vi "Filtered analysis.vi"() -> (5 "Plug in titles":string[](array[string]), 7 "Plug in values":string[](array[string]))   [LabVIEW 2011]
uses:
  <vilib>/Analysis/3filter.llb/Filter Passband Type.ctl
  Globals/Meas_global.vi
  <vilib>/Analysis/3filter.llb/Zero Phase Filter (Cascade, DBL).vi
  <vilib>/Analysis/NI_AALBase.lvlib
panel:
  out "XY Graph 5":cluster{"Time (ms)":dbl[], "Eng Values":dbl[]}[](graph)
  in  "Cutoff frequency (Hz)":dbl=50.0
  out "uw/u'w'":dbl
  out "u^2 4":dbl
  out "U 4":dbl
  out "u^2 3":dbl
  out "U 3":dbl
  out "XY Graph 4":cluster{"Time (ms)":dbl[], "Eng Values":dbl[]}[](graph)
  out "XY Graph 3":cluster{"Time (ms)":dbl[], "Eng Values":dbl[]}[](graph)
  out "uw/u'w' Filtered":dbl
  out "u^2 Filtered":dbl
  out "U filtered":dbl
  out "u^2 filtered":dbl
  out "U filtered":dbl
  in  "Invert values?":bool
  in  "Filter 2nd Instrument data?":bool
  in  "Freq Cutoff Inst 2":dbl=100.0
  in  "Freq Cutoff Inst 1":dbl=100.0
  in  "Filter 1st Instrument Data?":bool
  out "Time for max corr coeff":dbl
  out "Max corr coeff":dbl
  in  "Start point":dbl
  in  "Time step":dbl
  in  "Input own variables?":bool=TRUE
  out "Inst name 2":string
  out "Inst name":string
  out "Start point":dbl
  out "XY Graph 2":cluster{dbl[], dbl[]}(graph)
  out "Time step":dbl
  in  "Number of estimates":i32
  out "XY Graph":cluster{"Time (ms)":dbl[], "Eng Values":dbl[]}[](graph)
  in  "Instrumnt 2":i32=1
  in  "Instrument 1":i32
  # "Time lag"
  # "Correlation"
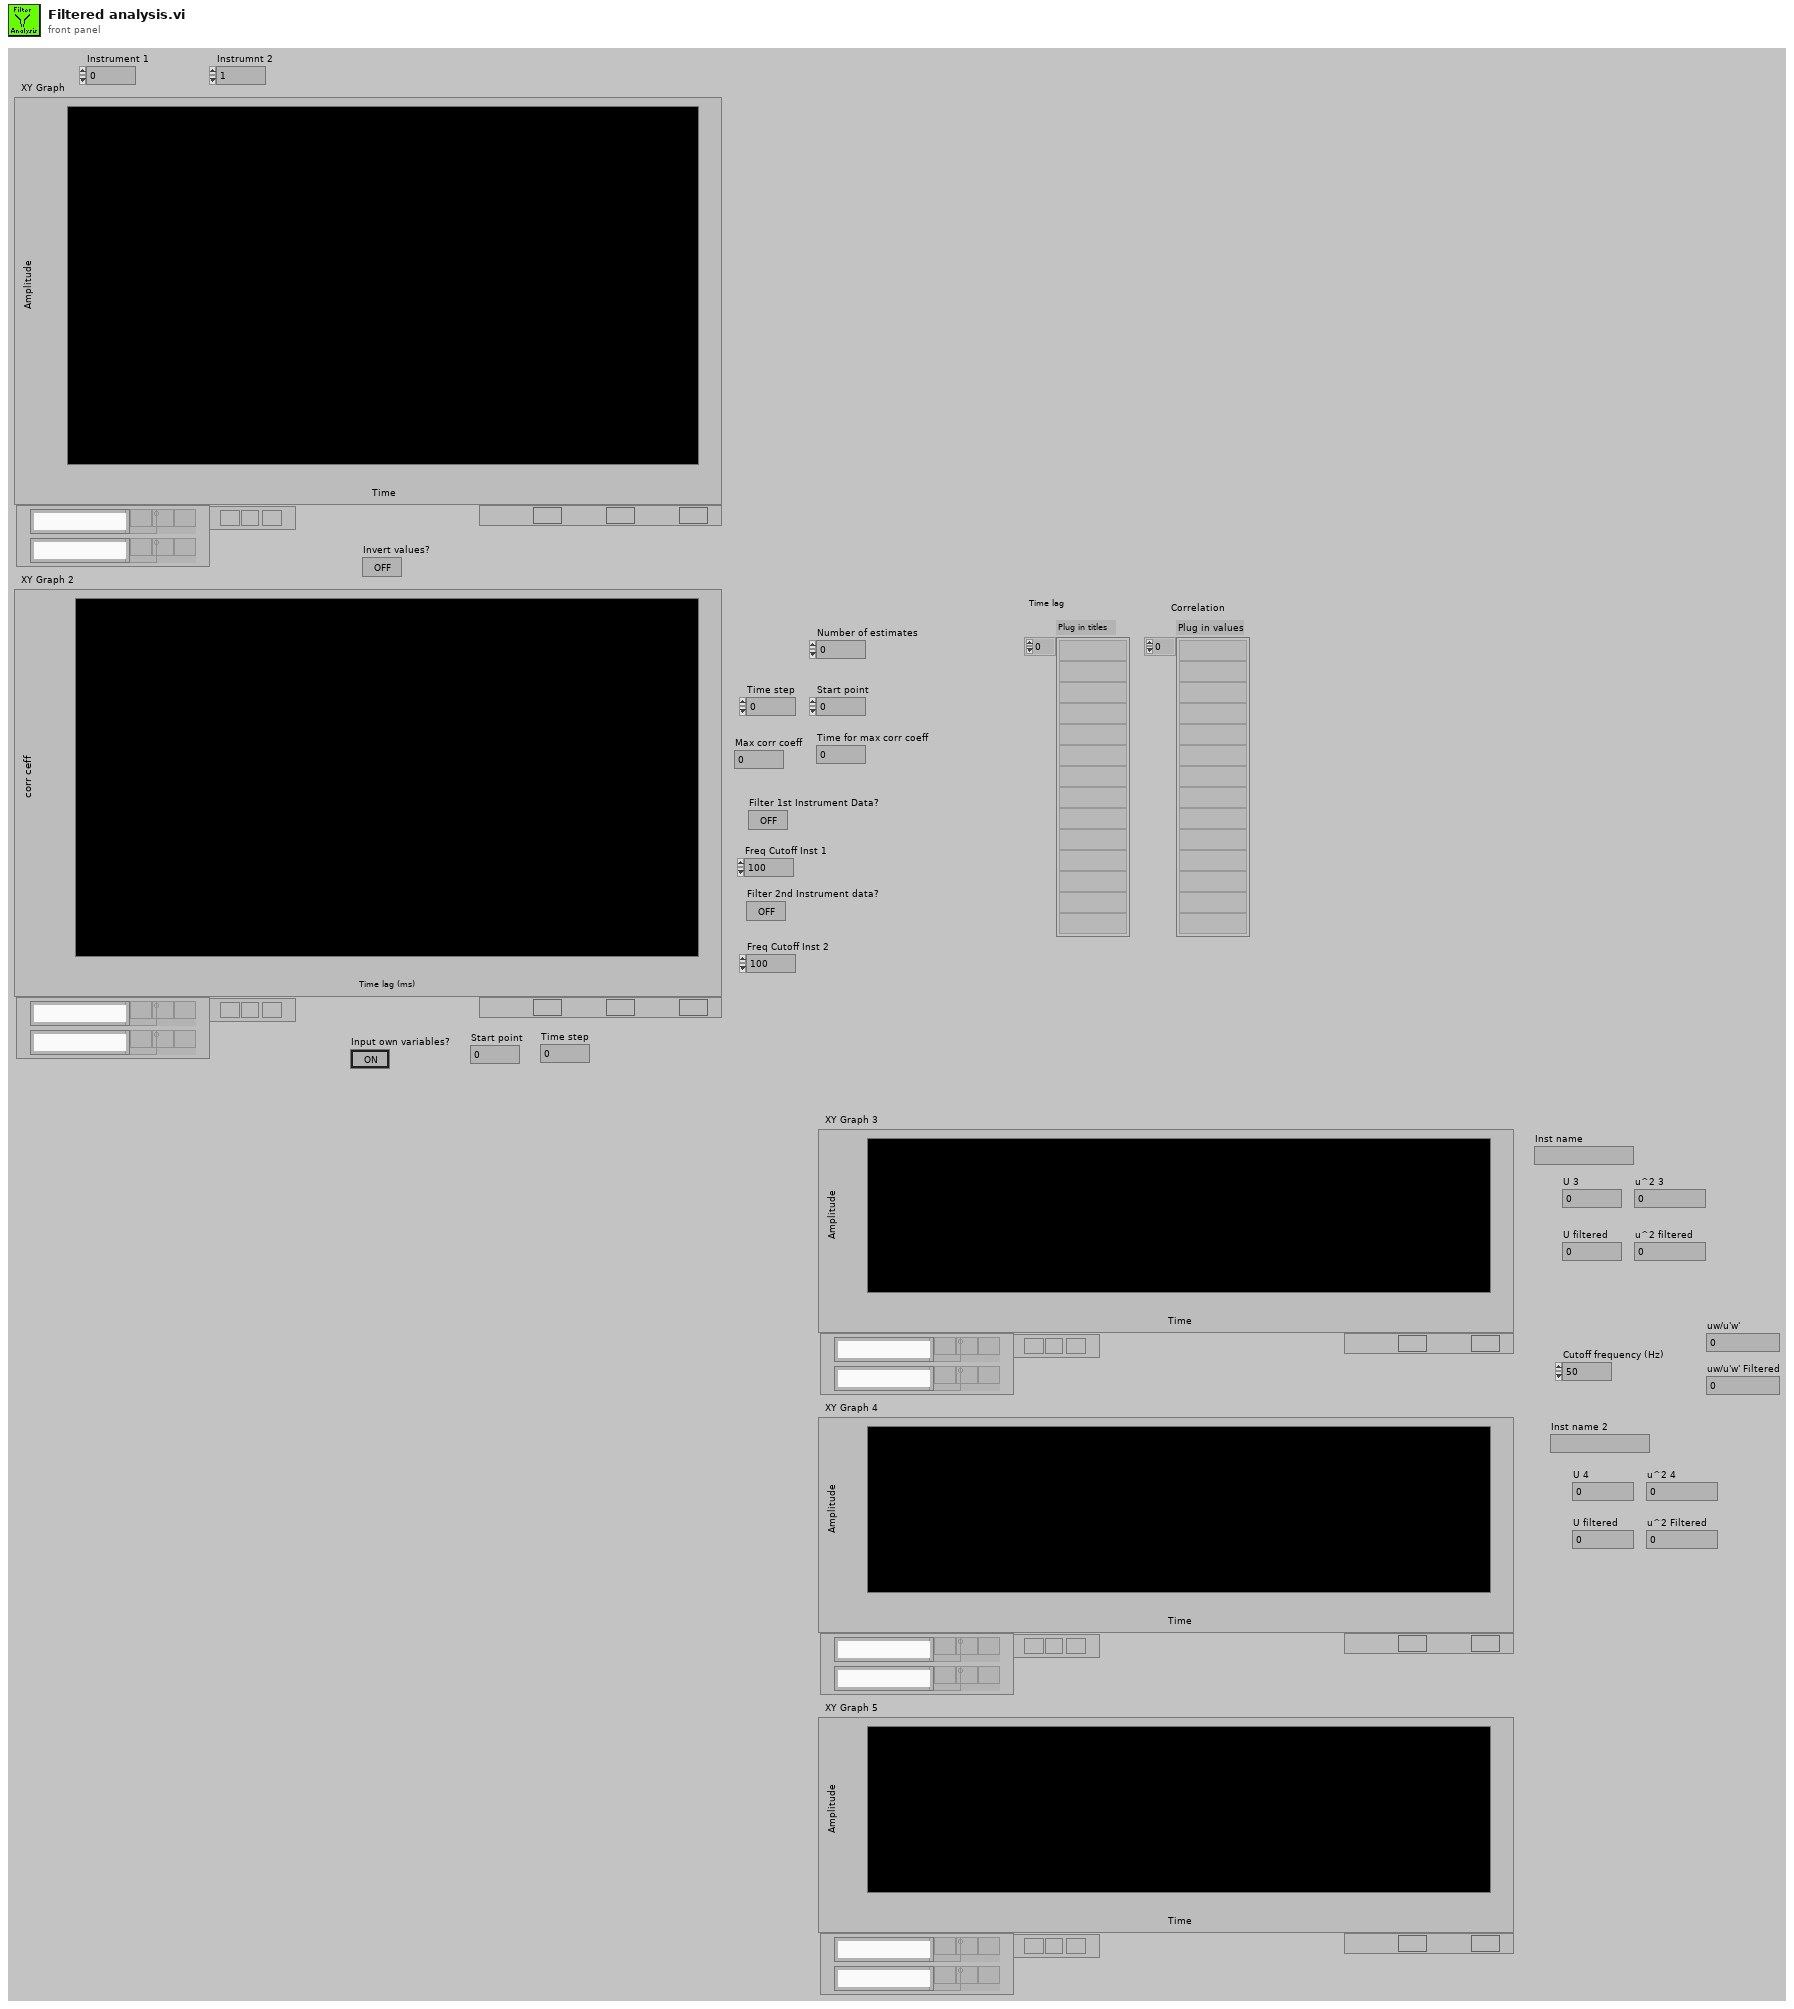
[diagram p1: front panel]
types:
  T1 = typedef "Analysis_info_cluster.ctl" = cluster{"Colour":u32, "Inst type":T2, "Inst name":string, "Symbol":string, "Code name":string, "Extra Info":string, "Inst Array":T3, "Extra Titles":string[], "Extra Values":string[], "Eng Values":dbl[], "Time (ms)":dbl[], "Voltage":dbl[], "U":dbl, "u^2":dbl, "u^3":dbl, "u^4":dbl, "Skew_u":dbl, "Kurt_u":dbl, "Sd Error in Mean":dbl, "% u'/U":dbl, "X":dbl, "Y":dbl, "Z":dbl, "Spectra":T4, "Autocorrelation":T4, "Timescale integral to 25%":dbl, "Sd Error in Variance":dbl, "Calib File":path, "Calib Constants":dbl[], "Histogram":T4, "Output Position":bool, "Full Stats":bool, "Weighting":dbl[], "Av Sampling Rate":dbl, "Av No of Samples":dbl, "Total Meas Time (s)":dbl}
  T2 = typedef "Inst_type.ctl" = enum16{"Propeller anemometer", "Raw voltage", "Pressure Transducer", "Pitot-static tube", "Preston tube", "Hot wire", "Cross wire 1", "Cross wire 2", "Generic Linear", "Generic Polynomial", "Generic BackPoly", "Fast FID", "Thermocouple", "Cold wire", "Pulsed Wire", "LDA Vel", "LDA Tran time", "LDA Arr time"}
  T3 = typedef "Instrument_Array.ctl" = enum16{"PWA", "LDA", "Analogue"}
  T4 = typedef "XY_Plot_Cluster.ctl" = cluster{"First Name":string, "Second Name":string, "X axis name":string, "Y axis name":string, "X array":dbl[], "Y array":dbl[]}
  T5 = typedef "NI_AALBase.lvlib/Filter Passband Type.ctl" = enum32{"Lowpass", "Highpass", "Bandpass", "Bandstop"}
  T6 = cluster{"filter structure":enum32{"IIR 2nd Order", "IIR 4th Order"}, "Reverse Coefficients":dbl[], "Forward Coefficients":dbl[]}
  T7 = typedef "Correlation_cluster1.ctl" = cluster{"U inst":string, "uw":dbl, "u^2w":dbl, "uw^2":dbl, "uw/u'w'":dbl, "W inst":string, "uw^3":dbl, "u^3w":dbl, "u^2w^2":dbl, "Index U":i32, "Index W":i32}
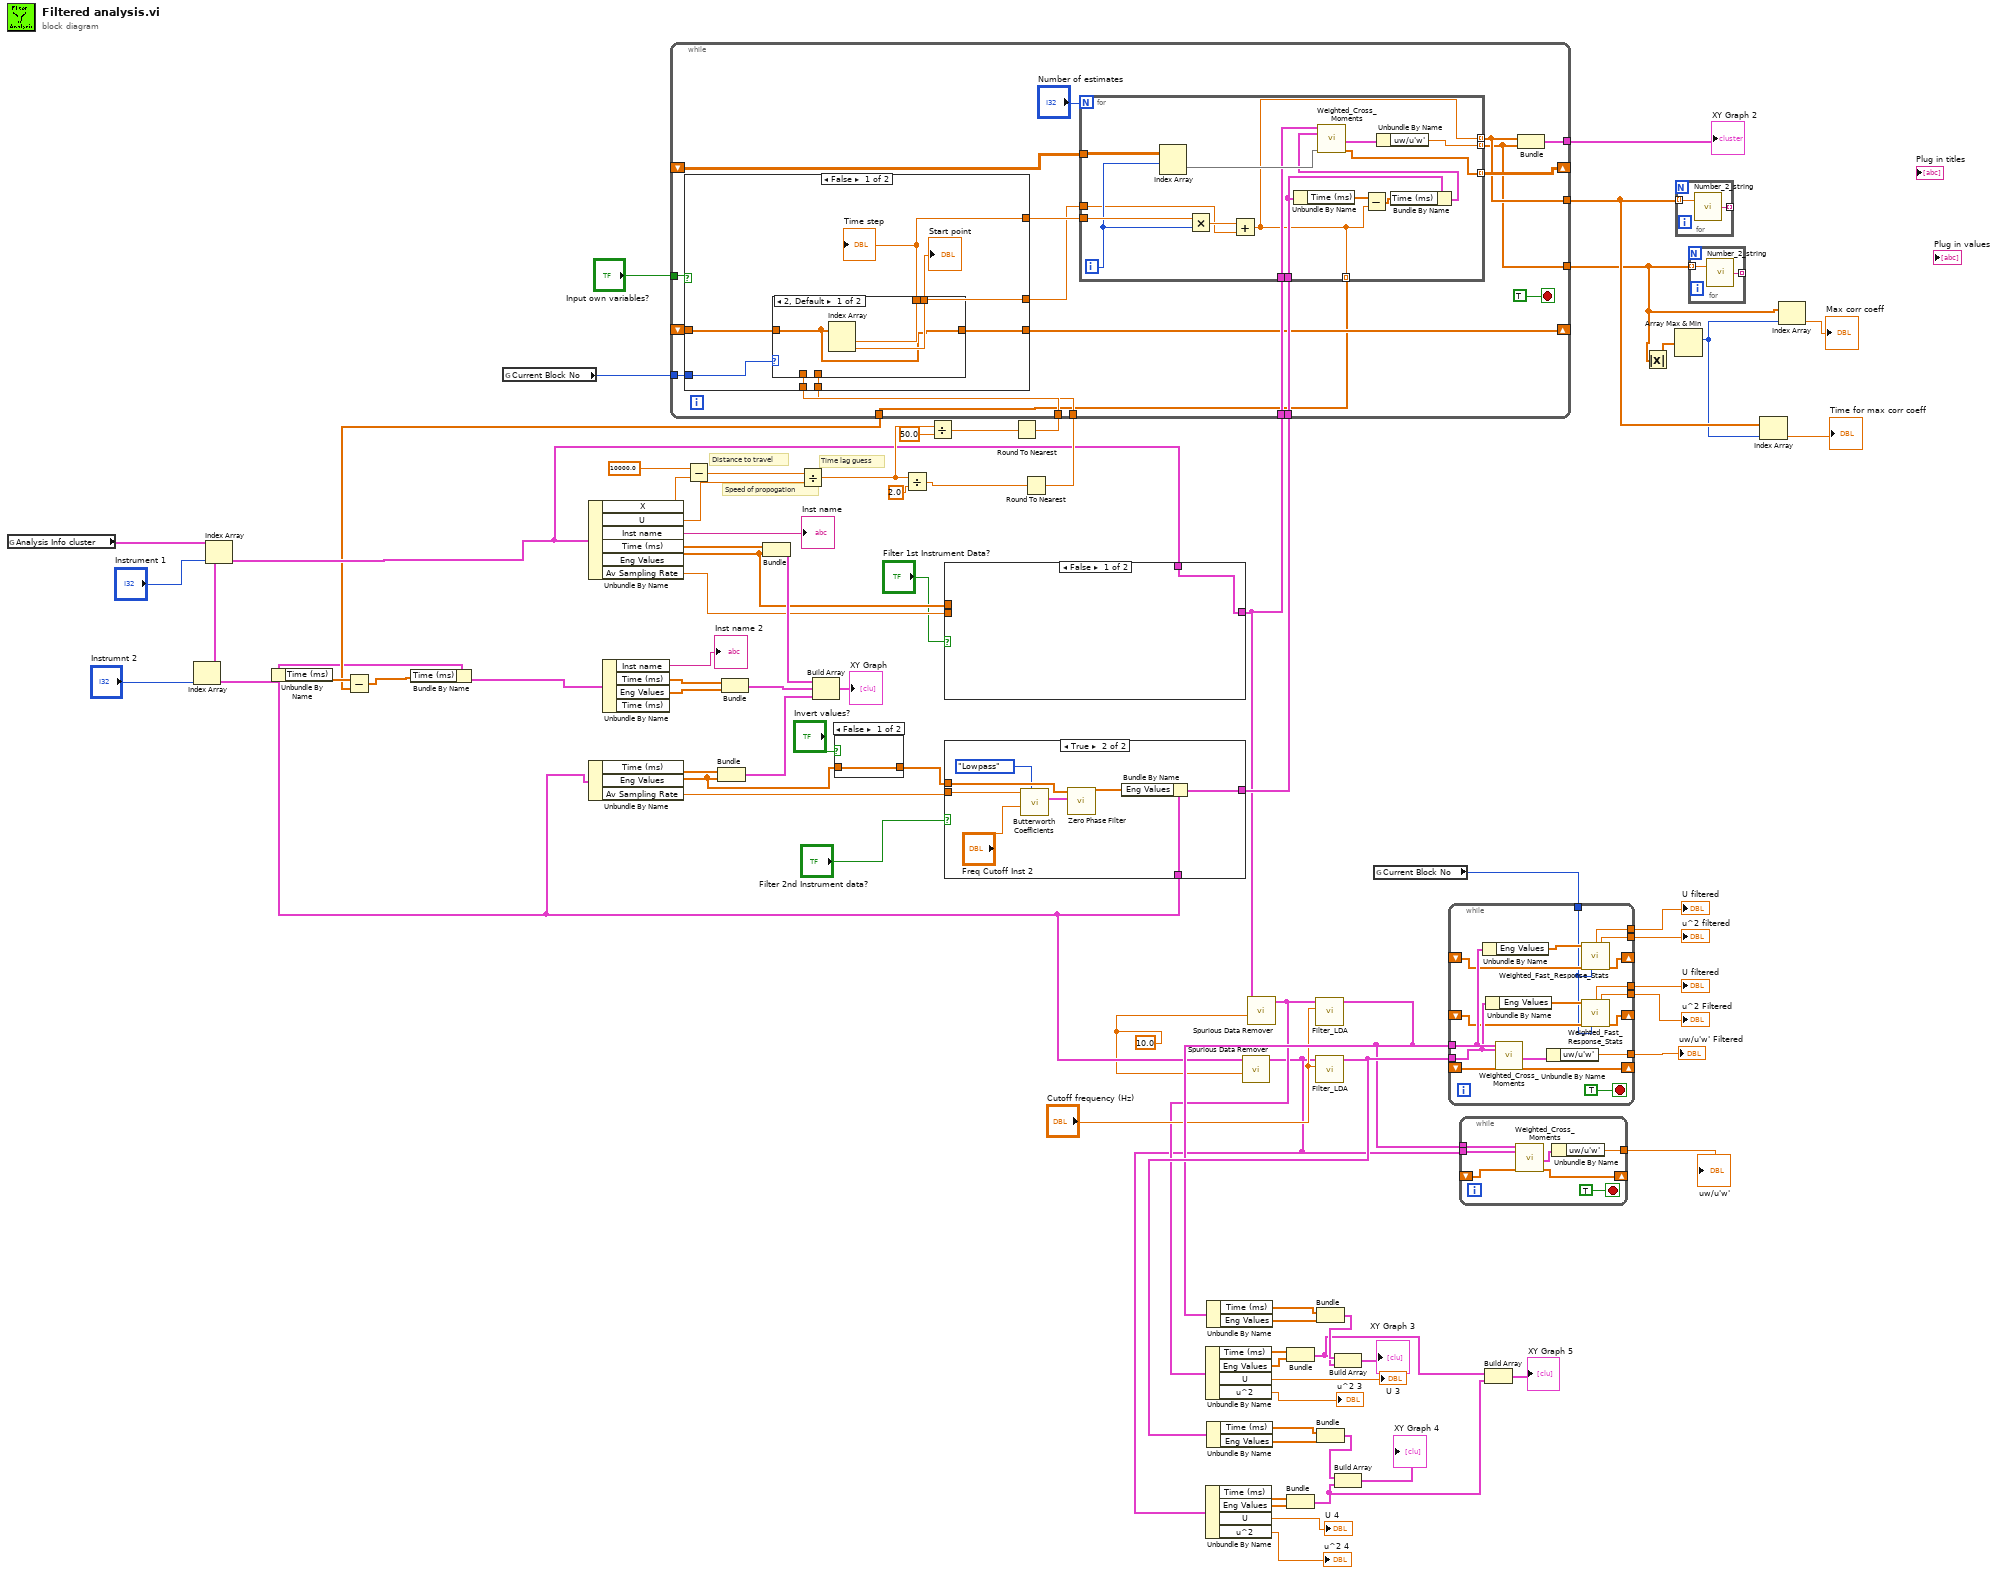
[diagram p0: block diagram]
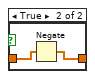
[diagram p2: hidden frame]
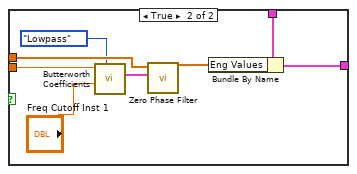
[diagram p4: hidden frame]
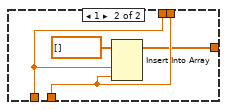
[diagram p5: hidden frame]
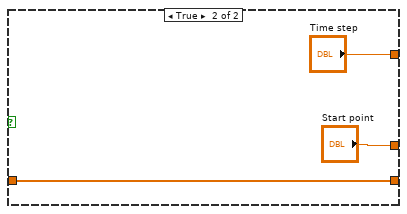
[diagram p6: hidden frame]
diagram:
  w1 = 10.0 ("St Dev threshold")
  # "Speed of propogation"
  # "Distance to travel"
  # "Time lag guess"
  n1 = global read "Meas_global.vi" "Analysis Info cluster"() -> (w71:T1[])
  n2 = Index Array(array=w71, index="Instrumnt 2") -> (element=w3:T1)
  n3 = Index Array(array=w71, index="Instrument 1") -> (element=w40:T1)
  n4 = Unbundle By Name(w3) -> ("Time (ms)"=w70:dbl[])
  n5 = global read "Meas_global.vi" "Current Block No"() -> (w58:i32)
  n6 = Unbundle By Name(w40) -> ("X"=w63:dbl, "U"=w65:dbl, "Inst name"=→"Inst name":string, "Time (ms)"=w75:dbl[], "Eng Values"=w50:dbl[], "Av Sampling Rate"=w49:dbl)
  n7 = Unbundle By Name(w3) -> ("Time (ms)"=w72:dbl[], "Eng Values"=w44:dbl[], "Av Sampling Rate"=w42:dbl)
  n8 = Subtract(x=10000.0, y=w63) -> (x-y=w62:dbl)
  n9 = Bundle("Time (ms)"=w72, "Eng Values"=w44) -> (w77:cluster{"Time (ms)":dbl[], "Eng Values":dbl[]})  [unwired: 1 in]
  n10 = Bundle("Time (ms)"=w75, "Eng Values"=w50) -> (w78:cluster{"Time (ms)":dbl[], "Eng Values":dbl[]})  [unwired: 1 in]
  n11 = Divide(x=w62, y=w65) -> (x/y=w60:dbl)
  n12 = case shown="False" "Invert values?" {
    tunnel: w44 -> [w82 w83]
    tunnel: [w82 w84] -> w43
    frame False {
    }
    frame True {
      n13 = Negate(x=w83) -> (-x=w84:dbl[])
    }
  }
  n14 = Divide(x=w60, y=2.0) -> (x/y=w55:dbl)
  n15 = Divide(x=w60, y=50.0) -> (x/y=w57:dbl)
  n16 = case shown="False" "Filter 1st Instrument Data?" {
    tunnel: w50 -> [_ w92]
    tunnel: w49 -> [_ w91]
    tunnel: w40 -> [w85 w89]
    tunnel: [w85 w88] -> w5
    frame False {
    }
    frame True {
      n17 = call <vilib>:"Butterworth Coefficients.vi"("filter type"=Filter_Passband_Type."Lowpass", "low cutoff freq: fl"="Freq Cutoff Inst 1", "sampling freq: fs"=w91) -> ("IIR Filter Cluster"=w93:T6)  [unwired: 7 in, 1 out]
      n18 = call-poly <vilib>:"Zero Phase Filter.vi"("IIR Filter Cluster"=w93, "X"=w92) -> ("Filtered X"=w90:dbl[])  [unwired: 8 in, 1 out]
      n19 = Bundle By Name(cluster=w89, "Eng Values"=w90) -> (w88:T1)
    }
  }
  n20 = case shown="True" "Filter 2nd Instrument data?" {
    tunnel: w43 -> [_ w101]
    tunnel: w42 -> [_ w100]
    tunnel: [w94 w98] -> w39
    tunnel: w3 -> [w94 w96]
    frame False {
    }
    frame True {
      n21 = call <vilib>:"Butterworth Coefficients.vi"("filter type"=Filter_Passband_Type."Lowpass", "low cutoff freq: fl"="Freq Cutoff Inst 2", "sampling freq: fs"=w100) -> ("IIR Filter Cluster"=w102:T6)  [unwired: 7 in, 1 out]
      n22 = call-poly <vilib>:"Zero Phase Filter.vi"("IIR Filter Cluster"=w102, "X"=w101) -> ("Filtered X"=w99:dbl[])  [unwired: 8 in, 1 out]
      n23 = Bundle By Name(cluster=w96, "Eng Values"=w99) -> (w98:T1)
    }
  }
  n24 = Round To Nearest(number=w57) -> (nearest integer value=w56:dbl)
  n25 = Round To Nearest(number=w55) -> (nearest integer value=w54:dbl)
  n26 = while {
    tunnel: w5 -> [w120]
    tunnel: w39 -> [w119]
    shift-right: [w117] -> _
    shift-left: _ -> [w116]
    tunnel: [w115] -> w68
    tunnel: [w113] -> w52
    tunnel: [w106] -> w36
    tunnel: w56 -> [w111]
    tunnel: w58 -> [w112]
    tunnel: w54 -> [w110]
    shift-right: [w109] -> _
    shift-left: _ -> [w108]
    tunnel: "Input own variables?" -> [w105]
    tunnel: [w103] -> w38
    stop <- TRUE stop-if-true
    n27 = case shown="False" w105 {
      tunnel: w112 -> [w127 _]
      tunnel: w111 -> [w126 _]
      tunnel: w110 -> [w125 _]
      tunnel: [w124 w135] -> w109
      tunnel: w108 -> [w123 w135]
      tunnel: [w122 "Start point"] -> w104
      tunnel: [w121 "Time step"] -> w107
      frame False {
        n28 = case shown="2, Default" w127 {
          tunnel: w126 -> [_ w133]
          tunnel: [w130 w133] -> w121
          tunnel: [w129 w134] -> w122
          tunnel: w125 -> [_ w134]
          tunnel: [w128 w132] -> w124
          tunnel: w123 -> [w128 _]
          frame 2, Default {
            n29 = Index Array(array=w128) -> (element #1=w130:dbl, element #2=w129:dbl)  [unwired: 2 in]
          }
          frame 1 {
            n30 = Insert Into Array(array=dbl[] [], new element #1=w133, new element #2=w134) -> (w132:dbl[])  [unwired: 1 in]
          }
        }
        "Time step" <- w121
        "Start point" <- w122
      }
      frame True {
      }
    }
    n31 = for {
      N: "Number of estimates" -> [_]
      tunnel: w120 -> [w146]
      tunnel: w119 -> [w142]
      tunnel: w107 -> [w152]
      tunnel: [w150] -> w117 mode=indexing
      tunnel: w116 -> [w149]
      tunnel: [w138] -> w113 mode=indexing
      tunnel: [w147] -> w106 mode=indexing
      tunnel: w104 -> [w139]
      tunnel: [w138] -> w103 mode=indexing
      i -> [w141]
      n32 = Index Array(array=w149, index (row)=w141) -> (element=w151:dbl[])  [unwired: 1 in]
      n33 = Multiply(x=w152, y=w141) -> (x*y=w140:dbl)
      n34 = Add(x=w140, y=w139) -> (x+y=w138:dbl)
      n35 = Unbundle By Name(w142) -> ("Time (ms)"=w145:dbl[])
      n36 = Subtract(x=w145, y=w138) -> (x-y=w144:dbl[])
      n37 = Bundle By Name(cluster=w142, "Time (ms)"=w144) -> (w143:T1)
      n38 = call "Weighted_Cross_Moments.vi"("Cluster 1"=w146, "Cluster 2"=w143, "Shift in"=w151) -> ("output cluster"=w148:T7, "Shift out"=w150:dbl[])  [unwired: 15 in]
      n39 = Unbundle By Name(w148) -> ("uw/u'w'"=w147:dbl)
    }
    n40 = Bundle(w113, w106) -> (w115:cluster{dbl[], dbl[]})  [unwired: 1 in]
  }
  "XY Graph 2" <- w68
  n41 = Subtract(x=w70, y=w38) -> (x-y=w69:dbl[])
  n42 = Bundle By Name(cluster=w3, "Time (ms)"=w69) -> (w41:T1)
  n43 = Unbundle By Name(w41) -> ("Inst name"=→"Inst name 2":string, "Time (ms)"=w74:dbl[], "Eng Values"=w73:dbl[])  [unwired: 1 out]
  n44 = Bundle("Time (ms)"=w74, "Eng Values"=w73) -> (w79:cluster{"Time (ms)":dbl[], "Eng Values":dbl[]})  [unwired: 1 in]
  n45 = Build Array(w78, w79, w77) -> (→"XY Graph":cluster{"Time (ms)":dbl[], "Eng Values":dbl[]}[])
  n46 = call "Spurious Data Remover.vi"("St Dev threshold"=w1, "Cluster 1"=w3) -> ("Cluster 1 Spurious points removed"=w2:T1)  [unwired: 9 in]
  n47 = Unbundle By Name(w2) -> ("Time (ms)"=w20:dbl[], "Eng Values"=w21:dbl[], "U"=→"U 4":dbl, "u^2"=→"u^2 4":dbl)
  n48 = call "Spurious Data Remover.vi"("St Dev threshold"=w1, "Cluster 1"=w5) -> ("Cluster 1 Spurious points removed"=w4:T1)  [unwired: 9 in]
  n49 = Unbundle By Name(w4) -> ("Time (ms)"=w26:dbl[], "Eng Values"=w16:dbl[], "U"=→"U 3":dbl, "u^2"=→"u^2 3":dbl)
  n50 = Bundle("Time (ms)"=w26, "Eng Values"=w16) -> (w8:cluster{"Time (ms)":dbl[], "Eng Values":dbl[]})  [unwired: 1 in]
  n51 = Bundle("Time (ms)"=w20, "Eng Values"=w21) -> (w7:cluster{"Time (ms)":dbl[], "Eng Values":dbl[]})  [unwired: 1 in]
  n52 = call "Filter_LDA.vi"("Cutoff frequency (Hz)"="Cutoff frequency (Hz)", "Cluster in"=w4) -> ("Cluster Out"=w11:T1)  [unwired: 6 in]
  n53 = Unbundle By Name(w11) -> ("Time (ms)"=w28:dbl[], "Eng Values"=w27:dbl[])
  n54 = call "Filter_LDA.vi"("Cutoff frequency (Hz)"="Cutoff frequency (Hz)", "Cluster in"=w2) -> ("Cluster Out"=w17:T1)  [unwired: 6 in]
  n55 = Unbundle By Name(w17) -> ("Time (ms)"=w18:dbl[], "Eng Values"=w19:dbl[])
  n56 = Bundle("Time (ms)"=w28, "Eng Values"=w27) -> (w24:cluster{"Time (ms)":dbl[], "Eng Values":dbl[]})  [unwired: 1 in]
  n57 = Bundle("Time (ms)"=w18, "Eng Values"=w19) -> (w23:cluster{"Time (ms)":dbl[], "Eng Values":dbl[]})  [unwired: 1 in]
  n58 = Build Array(w24, w8) -> (→"XY Graph 3":cluster{"Time (ms)":dbl[], "Eng Values":dbl[]}[])
  n59 = Build Array(w23, w7) -> (→"XY Graph 4":cluster{"Time (ms)":dbl[], "Eng Values":dbl[]}[])
  n60 = global read "Meas_global.vi" "Current Block No"() -> (w34:i32)
  n61 = while {
    tunnel: w11 -> [w167]
    tunnel: w17 -> [w166]
    shift-right: [w169] -> _
    shift-left: _ -> [w170]
    tunnel: [w163] -> w29
    tunnel: [w162] -> w31
    tunnel: [w161] -> w30
    tunnel: [w160] -> w33
    tunnel: [w159] -> w32
    shift-right: [w155] -> _
    shift-left: _ -> [w156]
    shift-right: [w157] -> _
    shift-left: _ -> [w158]
    tunnel: w34 -> [w154]
    stop <- TRUE stop-if-true
    n62 = Unbundle By Name(w167) -> ("Eng Values"=w165:dbl[])
    n63 = Unbundle By Name(w166) -> ("Eng Values"=w164:dbl[])
    n64 = call "Weighted_Cross_Moments.vi"("Cluster 1"=w167, "Cluster 2"=w166, "Shift in"=w170) -> ("output cluster"=w168:T7, "Shift out"=w169:dbl[])  [unwired: 15 in]
    n65 = Unbundle By Name(w168) -> ("uw/u'w'"=w163:dbl)
    n66 = call "Weighted_Fast_Response_Stats.vi"("U"=w165, "Shift in"=w158, "Block No"=w154) -> ("U"=w160:dbl, "u^2"=w159:dbl, "Shift out"=w157:dbl[])  [unwired: 5 in, 5 out]
    n67 = call "Weighted_Fast_Response_Stats.vi"("U"=w164, "Shift in"=w156, "Block No"=w154) -> ("U"=w162:dbl, "u^2"=w161:dbl, "Shift out"=w155:dbl[])  [unwired: 5 in, 5 out]
  }
  "U filtered" <- w33
  "u^2 filtered" <- w32
  "U filtered" <- w31
  "u^2 Filtered" <- w30
  "uw/u'w' Filtered" <- w29
  n68 = while {
    tunnel: w11 -> [w177]
    tunnel: w2 -> [w176]
    shift-right: [w174] -> _
    shift-left: _ -> [w175]
    tunnel: [w172] -> w10
    stop <- TRUE stop-if-true
    n69 = call "Weighted_Cross_Moments.vi"("Cluster 1"=w177, "Cluster 2"=w176, "Shift in"=w175) -> ("output cluster"=w173:T7, "Shift out"=w174:dbl[])  [unwired: 15 in]
    n70 = Unbundle By Name(w173) -> ("uw/u'w'"=w172:dbl)
  }
  "uw/u'w'" <- w10
  n71 = Build Array(w8, w7) -> (→"XY Graph 5":cluster{"Time (ms)":dbl[], "Eng Values":dbl[]}[])
  n72 = Absolute Value(x=w36) -> (abs(x)=w46:dbl[])
  n73 = Array Max & Min(array=w46) -> (max index (indices)=w37:i32)  [unwired: 3 out]
  n74 = for {
    tunnel: w52 -> [w178] mode=indexing
    tunnel: [w179] -> _ mode=indexing
    n75 = call "Number_2_string.vi"("number"=w178) -> ("String"=w179:string)  [unwired: 1 in]
  }
  n76 = for {
    tunnel: w36 -> [w180] mode=indexing
    tunnel: [w181] -> _ mode=indexing
    n77 = call "Number_2_string.vi"("number"=w180) -> ("String"=w181:string)  [unwired: 1 in]
  }
  n78 = Index Array(array=w52, index=w37) -> (element=→"Time for max corr coeff":dbl)
  n79 = Index Array(array=w36, index=w37) -> (element=→"Max corr coeff":dbl)
